vi "data entry limit.vi"(8 "error in (no error)":errorcluster caption="에러 입력(에러 없음)", 11 "Waveform Obj 입력":refnum<class "Waveform Gen.lvclass">) -> (0 "error out":errorcluster caption="에러 출력", 3 "Waveform Obj 출력":refnum<class "Waveform Gen.lvclass">)   [LabVIEW 2020, in "Waveform Gen.lvclass"]
uses:
  Waveform Gen.lvclass
  Waveform Gen.lvclass/Waveform Gen.ctl
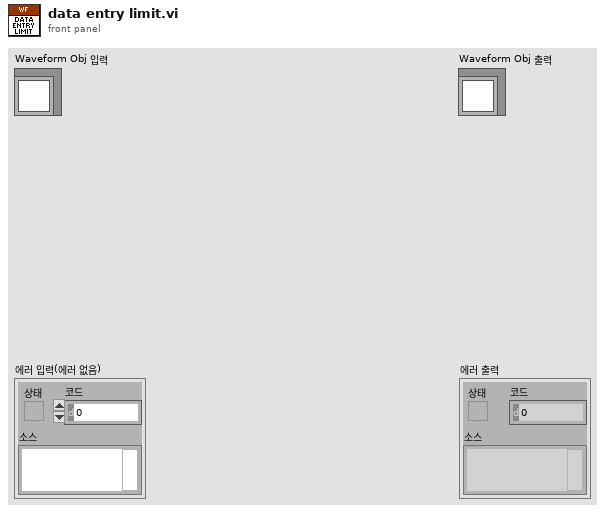
[diagram p1: front panel]
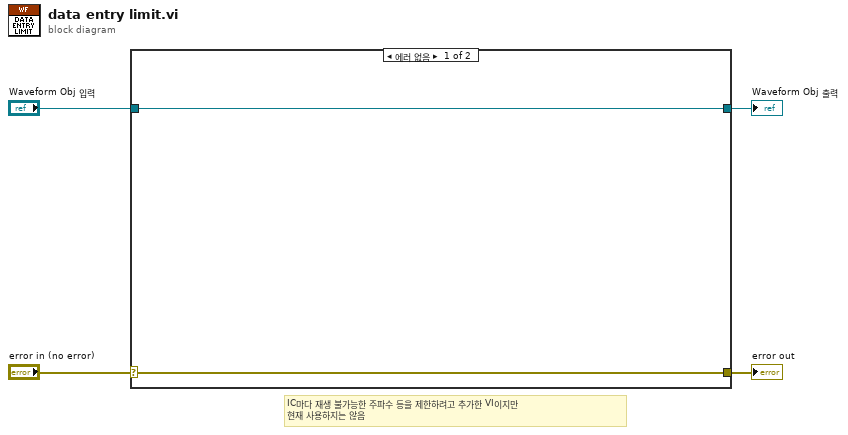
[diagram p0: block diagram]
diagram:
  # "IC마다 재생 불가능한 주파수 등을 제한하려고 추가한 VI이지만\n현재 사용하지는 않음"
  n1 = case shown="에러 없음" "error in (no error)" {
    selector: "error in (no error)" -> [w5 w8]
    tunnel: [w5 w8] -> w3
    tunnel: [w6 w7] -> w1
    tunnel: "Waveform Obj 입력" -> [w6 w7]
    frame No Error {
    }
    frame Error {
    }
  }
  "error out" <- w3
  "Waveform Obj 출력" <- w1
